vi "MainDAQUse.vi"() -> ()   [LabVIEW 2023]
uses:
  <vilib>/express/express signal manip/GetorSetDDTAttributes/Shared VIs/TimeType.ctl
  <vilib>/DAQmx/read.llb/DAQmx Read (Analog 2D DBL NChan NSamp).vi
  5948bca3-3d14-40bf-9fbb-2ba5c3eee3bd.vi
  <vilib>/Analysis/baseanly.llb/Mean (DBL).vi
  faa81322-6883-41b3-8229-1eb533283c0b.vi
  <extravilib>/ChannelInstances/Tag-bool/Read With Abort.vi
  <extravilib>/ChannelInstances/Tag-bool/Write With Abort.vi
  <extravilib>/ChannelInstances/Tag-bool/Instantiate.vi
  <vilib>/DAQmx/miscellaneous.llb/DAQmx Fill In Error Info.vi
  <extravilib>/ChannelInstances/Tag-bool/EndpointRead.vi
  <vilib>/express/express signal manip/GetorSetDDTAttributes/Shared VIs/TimeMode Enum to Boolean.vi
  <vilib>/express/express shared/transition.llb/Dynamic To Waveform Array.vi
  <vilib>/express/express signal manip/GetorSetDDTAttributes/Set DDT Attributes/SetT0.vi
  <vilib>/express/express shared/transition.llb/Waveform Array To Dynamic.vi
  <extravilib>/ChannelInstances/Tag-bool/Endpoint.vi
  <vilib>/express/express signal manip/GetorSetDDTAttributes/Set DDT Attributes/Set DDT Properties.xnode
  <extravilib>/ChannelInstances/Tag-bool.lvlib
  <vilib>/ptbypt/NI_PtbyPt.lvlib
  <vilib>/Analysis/NI_AALBase.lvlib
  <vilib>/express/express signal manip/GetorSetDDTAttributes/Shared VIs/GetSetShared.lvlib
panel:
  out "Prueba de frecuencia":dynamicdata(graph)
  out "Array":dbl[][](array[numeric])
  out "dt":dbl
  in  "?":T1(tab)
  out "Valor numérico voltaje ACS sin offset":dbl
  out "Signal Frequency":dbl(graph)
  out "Stable RPM measurement?":bool
  in  "R de carga [Ohm]":dbl
  in  "Omega Nominal [RPM]":dbl
  in  "Voltage Threshold":dbl=0.5
  in  "Number of magnets":dbl=1.0
  out "Omega [RPM]":dbl(knob) scale=0.0..2000.0
  out "Voltaje Diodo RMS [V]":dbl(knob) scale=0.0..20.0
  out "Potencia [W]":dbl(knob) scale=0.0..20.0
  out "Voltaje ACS RMS [V]":dbl(knob) scale=0.0..20.0
  in  "Button":bool
  out "Signal\nFrequency (Hz)":dbl
  in  "?":bool
  in  "Button 2":bool
  out "Python Error Status":errorcluster
  in  "Filename":path=path "C:/Users/johan/OneDrive - Estudiantes ITCR/TEC/ProyectodeGraduacion/LabEolicaControl/rawdata.txt"
  out "Corriente ACS RMS [mA]":dbl(knob) scale=0.0..20.0
  out "Valor numérico\nCorriente [mA]":dbl
  out "V Gen RMS [V]":dbl(knob) scale=0.0..20.0
  in  "R1 [Ohm]":dbl=1.0
  in  "R2 [Ohm]":dbl=1.0
  in  "Offset del ACS [V]":dbl=1.0
  in  "Sensibilidad ACS [mV/A]":dbl=1.0
  out "Voltaje diodo [V]":dynamicdata(graph)
  out "Sensor ACS [V]":dynamicdata(graph)
  out "Senal Pulsos":dynamicdata(graph)
  out "Sensor Hall [V]":dynamicdata(graph)
  # "Lab Setup"
  # "Data Monitoring"
  # "Datos para el DAQ"
  # "Condiciones del punto de medida"
  # "File I/O"
  # "Post Processing"
  # "About:"
  # "Software Requirements:"
  # "This measuring system was designed for data acquisition of \npower, angular speed, and resistance data for small scale HAWT \nand possibly VAWT. These turbines are being researched and \ndeveloped at LIENE (Laboratorio de Investigación en Energía Eólica) \nat ITCR. \n\nThis software acquires data and performs post processing to obtain \npower graphs and surfaces and data tables for further analysis. It uses \nLabView for DAQ and integrated Python scripts to post process and \ngraph data."
  # "Python 3.6 with the following packages:\n-- NumPy\n-- Plotly"
  # "Programmer:"
  # "This software was designed and programmed by: \n-- Johansell Villalobos Cubillo & Mauricio Bolivar Gonzalez: \n         Engineering Physics students"
  # "DAQ Equipment: NI-USB-6000"
  # "The equipment pinout diagram is shown below and the pins are used as follows: \n\nAl 0 -- Hall effect sensor\nAl 1-- Voltage sensor\nAl 2 -- ACS712 10A current sensor\nAl GND -- common ground"
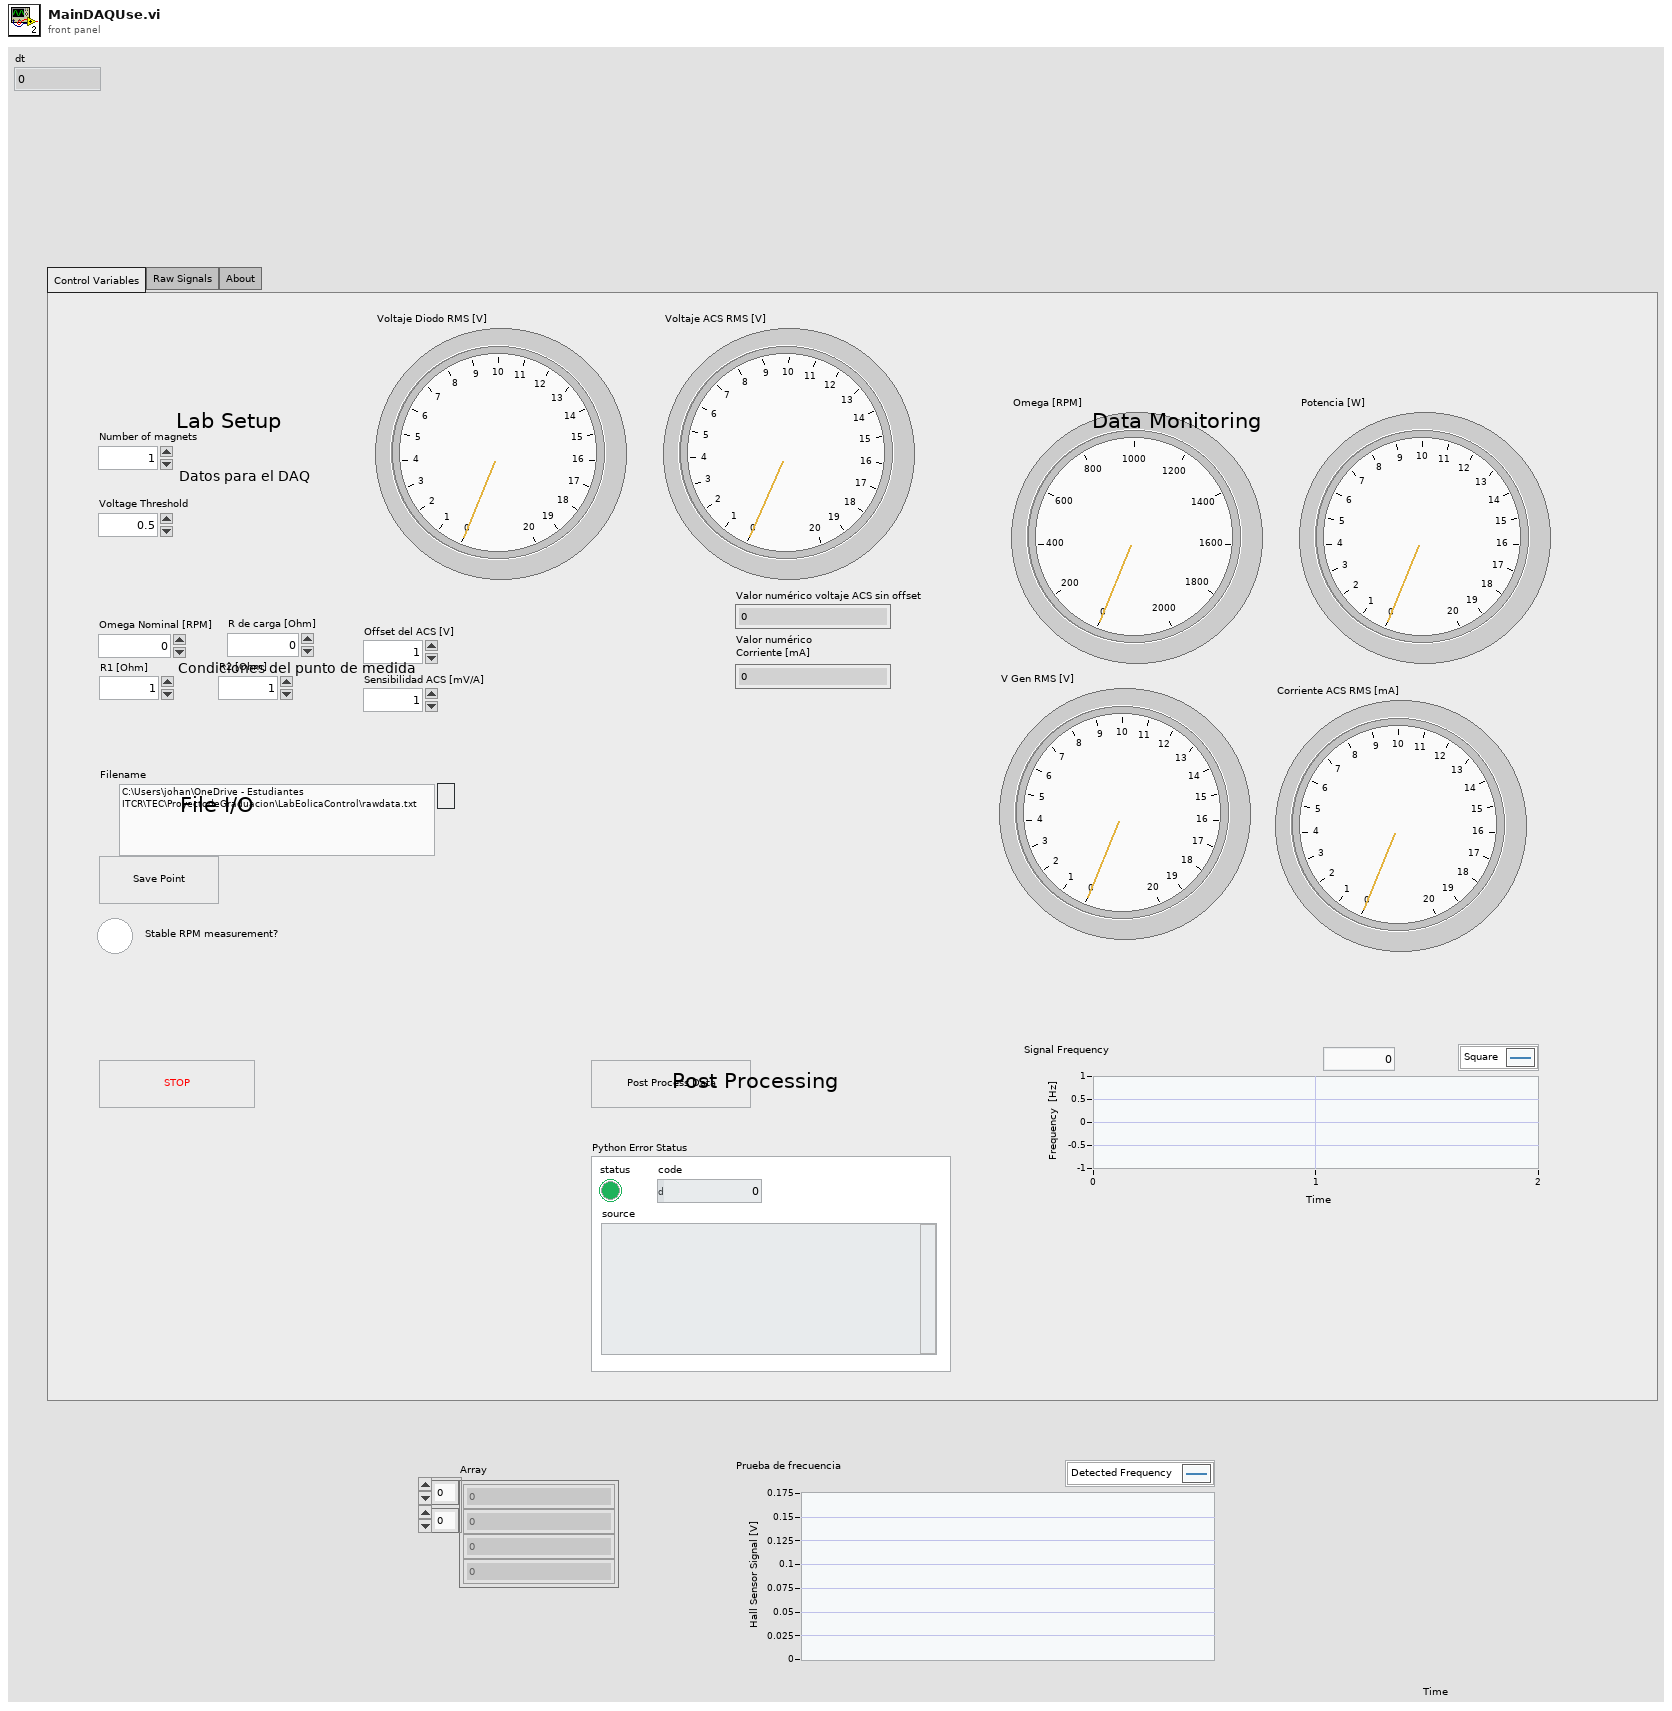
[diagram p1: front panel]
types:
  T1 = enum32{"Control Variables", "Raw Signals", "About"}
  T2 = typedef "Tag-bool.lvlib/))Channel.ctl" = refnum<queue>
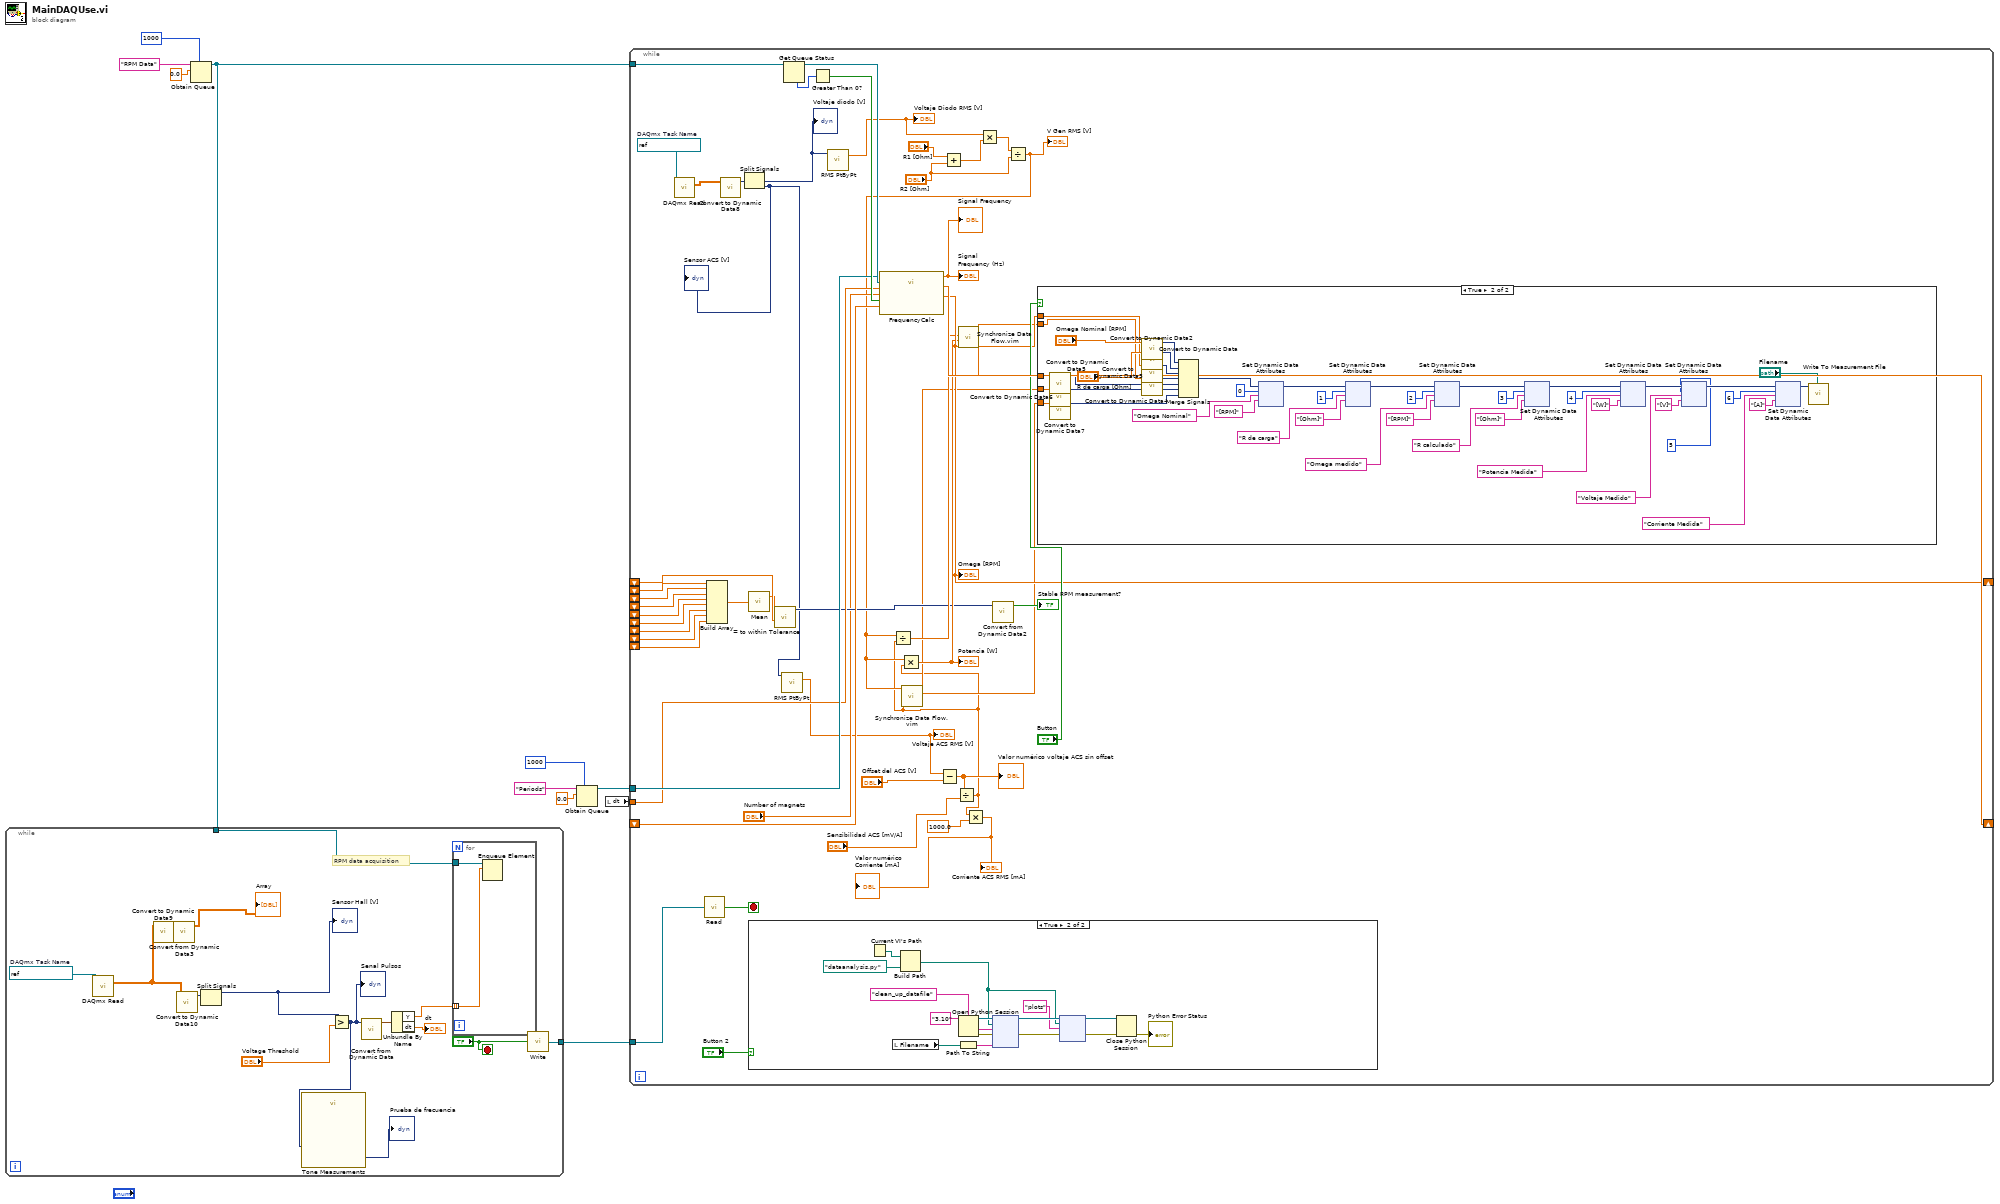
[diagram p0: block diagram]
diagram:
  n1 = Obtain Queue(max queue size (-1, unlimited)=1000 ("max queue size\n(-1, unlimited)"), name (unnamed)="RPM Data" ("name\n(unnamed)"), element data type=0.0 ("data type\n(double)")) -> (queue out=w5:refnum<queue>)  [unwired: 2 in, 2 out]
  n2 = while {
    tunnel: w5 -> [w23]
    tunnel: [w21] -> w7
    stop <- "?" stop-if-true
    w17 = refnum<k21> "DAQ ACS2_0"  # DAQmx Task Name
    # "RPM data acquisition"
    n3 = call-poly <vilib>:"DAQmx Read.vi"("task/channels in"=w17) -> ("data"=w14:dbl[][])  [unwired: 12 in, 2 out]
    n4 = call "Convert to Dynamic Data9"("2D Array"=w14) -> ("Dynamic Data Type"=w16:dynamicdata)  [unwired: 3 in]
    n5 = call "Convert from Dynamic Data3"("Dynamic Data Type"=w16) -> ("Array"=→"Array":dbl[][])  [unwired: 3 in]
    n6 = call "Convert to Dynamic Data10"("2D Array"=w14) -> ("Dynamic Data Type"=w15:dynamicdata)  [unwired: 3 in]
    n7 = Split Signals(w15) -> (w12:dynamicdata)  [unwired: 3 in, 2 out]
    "Sensor Hall [V]" <- w12
    n8 = Greater?(x=w12, y="Voltage Threshold") -> (0:w11:dynamicdata)
    "Senal Pulsos" <- w11
    n9 = call "Tone Measurements"("Signals"=w11) -> ("Frequency"=→"Prueba de frecuencia":dynamicdata)  [unwired: 9 in, 1 out]
    n10 = call "Convert from Dynamic Data"("Dynamic Data Type"=w11) -> ("Waveform"=w25:waveform(dbl))  [unwired: 3 in]
    n11 = Unbundle By Name(w25) -> ("Y"=w24:dbl[], "dt"=→"dt":dbl)
    n12 = for {
      tunnel: w24 -> [w27] mode=indexing
      tunnel: w23 -> [w26]
      n13 = Enqueue Element(queue=w26, element=w27) -> ()  [unwired: 2 in, 3 out]
    }
    n14 = call <extravilib>:"Write.vi"("element"="?") -> ("channel"=w21:T2)  [unwired: 1 out]
  }
  n15 = Obtain Queue(max queue size (-1, unlimited)=1000 ("max queue size\n(-1, unlimited)"), name (unnamed)="Periods" ("name\n(unnamed)"), element data type=0.0 ("data type\n(double)")) -> (queue out=w1:refnum<queue>)  [unwired: 2 in, 2 out]
  n16 = local read "dt"() -> (w6:dbl)
  n17 = while {
    tunnel: w5 -> [w79]
    tunnel: w1 -> [w76]
    shift-right: [w74] -> _
    shift-left: _ -> [w75]
    tunnel: w6 -> [w71]
    tunnel: w7 -> [w72]
    shift-right: [w69] -> _
    shift-left: _ -> [w63]
    shift-left: _ -> [w64]
    shift-left: _ -> [w65]
    shift-left: _ -> [w66]
    shift-left: _ -> [w61]
    shift-left: _ -> [w52]
    shift-left: _ -> [w51]
    shift-left: _ -> [w50]
    shift-left: _ -> [w49]
    stop <- w73 stop-if-true
    w45 = refnum<k21> "DAQ ACS2_0"  # DAQmx Task Name
    n18 = call-poly <vilib>:"DAQmx Read.vi"("task/channels in"=w45) -> ("data"=w44:dbl[][])  [unwired: 12 in, 2 out]
    n19 = call <extravilib>:"Read.vi"("channel"=w72) -> ("element"=w73:bool)  [unwired: 1 in, 1 out]
    n20 = Build Array(w66, w65, w64, w63, w52, w51, w50, w49) -> (w62:dbl[])
    n21 = call "Convert to Dynamic Data8"("2D Array"=w44) -> ("Dynamic Data Type"=w42:dynamicdata)  [unwired: 3 in]
    n22 = Split Signals(w42) -> (w41:dynamicdata, w43:dynamicdata)  [unwired: 3 in, 1 out]
    "Sensor ACS [V]" <- w43
    "Voltaje diodo [V]" <- w41
    n23 = call-poly <vilib>:"Mean.vi"("X"=w62) -> ("mean"=w60:dbl)  [unwired: 1 out]
    n24 = case shown="True" "Button 2" {
      frame False {
      }
      frame True {
        n25 = Current VI's Path() -> (path=w88:path)
        n26 = local read "Filename"() -> (w91:path)
        n27 = Build Path(base path=w88, name or relative path=path "dataanalysis.py") -> (appended path=w85:path)
        n28 = Path To String(path=w91) -> (string=w92:string)
        n29 = Open Python Session(python version="3.10" ("Python version")) -> (session out=w93:refnum<k35>, error out=w94:errorcluster)  [unwired: 2 in]
        n30 = node(w93, w85, "clean_up_datafile" ("function name"), w94, w92) -> (w86:refnum<k35>, w83:errorcluster)  [unwired: 3 in, 2 out]
        n31 = node(w86, w85, "plots" ("function name"), w83) -> (w81:refnum<k35>, w82:errorcluster)  [unwired: 2 in, 2 out]
        n32 = Close Python Session(session in=w81, error in=w82) -> (11:→"Python Error Status":errorcluster)
      }
    }
    n33 = call "= to within Tolerance"("Constant Value to Compare Against"=w61, "Operand 1"=w60) -> ("Result"=w59:dynamicdata)  [unwired: 8 in, 1 out]
    n34 = call <vilib>:"RMS PtByPt.vi"("x"=w43) -> ("rms value"=w40:dbl)  [unwired: 3 in, 1 out]
    "Voltaje ACS RMS [V]" <- w40
    n35 = Get Queue Status(queue=w79) -> (queue out=w77:refnum<queue>, # elements in queue=w80:i32)  [unwired: 2 in, 6 out]
    n36 = Greater Than 0?(x=w80) -> (x > 0?=w78:bool)
    n37 = call <vilib>:"RMS PtByPt.vi"("x"=w41) -> ("rms value"=w30:dbl)  [unwired: 3 in, 1 out]
    "Voltaje Diodo RMS [V]" <- w30
    n38 = call "FrequencyCalc.vi"("Checkbox"=w78, "Number of teeth in gear"="Number of magnets", "Period\n(s) in"=w75, "dt"=w71, "queue in"=w77, "Queue in"=w76) -> ("Omega [RPM]"=w69:dbl, "Period\n(s) out"=w74:dbl, "Signal Frequency (Hz)"=→"Signal\nFrequency (Hz)" →"Signal Frequency":dbl)  [unwired: 2 in, 1 out]
    "Omega [RPM]" <- w69
    n39 = Subtract(x=w40, y="Offset del ACS [V]") -> (x-y=w37:dbl)
    "Valor numérico voltaje ACS sin offset" <- w37
    n40 = Add(x="R1 [Ohm]", y="R2 [Ohm]") -> (x+y=w34:dbl)
    n41 = Divide(x=w37, y="Sensibilidad ACS [mV/A]") -> (x/y=w28:dbl)
    n42 = Multiply(x=w28, y=1000.0) -> (x*y=→"Corriente ACS RMS [mA]" →"Valor numérico\nCorriente [mA]":dbl)
    n43 = Multiply(x=w30, y=w34) -> (x*y=w36:dbl)
    n44 = call "Convert from Dynamic Data2"("Dynamic Data Type"=w59) -> ("Scalar"=→"Stable RPM measurement?":bool)  [unwired: 3 in]
    n45 = Divide(x=w36, y="R2 [Ohm]") -> (x/y=w29:dbl)
    "V Gen RMS [V]" <- w29
    n46 = Divide(x=w29, y=w28) -> (x/y=w68:dbl)
    n47 = Multiply(x=w29, y=w28) -> (x*y=w67:dbl)
    "Potencia [W]" <- w67
    n48 = call "Synchronize Data Flow.vim"("input 2"=w28, "input 1"=w29) -> ("output 2"=w46:dbl, "output 1"=w47:dbl)  [unwired: 2 in, 2 out]
    n49 = call "Synchronize Data Flow.vim"("input 4"=w69, "input 3"=w67, "input 2"=w68) -> ("output 4"=w57:dbl, "output 3"=w55:dbl, "output 2"=w56:dbl)  [unwired: 1 in, 1 out]
    n50 = case shown="True" "Button" {
      tunnel: w57 -> [_ w134]
      tunnel: w56 -> [_ w135]
      tunnel: w55 -> [_ w130]
      tunnel: w47 -> [_ w108]
      tunnel: w46 -> [_ w107]
      frame False {
      }
      frame True {
        n51 = call "Convert to Dynamic Data5"("Double"=w130) -> ("Dynamic Data Type"=w131:dynamicdata)  [unwired: 3 in]
        n52 = call "Convert to Dynamic Data6"("Double"=w108) -> ("Dynamic Data Type"=w106:dynamicdata)  [unwired: 3 in]
        n53 = call "Convert to Dynamic Data7"("Double"=w107) -> ("Dynamic Data Type"=w105:dynamicdata)  [unwired: 3 in]
        n54 = call "Convert to Dynamic Data"("Double"="Omega Nominal [RPM]") -> ("Dynamic Data Type"=w137:dynamicdata)  [unwired: 3 in]
        n55 = call "Convert to Dynamic Data2"("Double"="R de carga [Ohm]") -> ("Dynamic Data Type"=w136:dynamicdata)  [unwired: 3 in]
        n56 = call "Convert to Dynamic Data3"("Double"=w134) -> ("Dynamic Data Type"=w133:dynamicdata)  [unwired: 3 in]
        n57 = call "Convert to Dynamic Data4"("Double"=w135) -> ("Dynamic Data Type"=w132:dynamicdata)  [unwired: 3 in]
        n58 = Merge Signals(w137, w136, w133, w132, w131, w106, w105) -> (w129:dynamicdata)
        n59 = xnode ("Set Dynamic Data Attributes")("Signals In"=w129, "Signal Index"=0, "Signal Name"="Omega Nominal", "Unit"="[RPM]") -> ("Signals Out"=w122:dynamicdata)  [unwired: 3 in, 1 out]
        n60 = xnode ("Set Dynamic Data Attributes")("Signals In"=w122, "Signal Index"=1, "Signal Name"="R de carga", "Unit"="[Ohm]") -> ("Signals Out"=w118:dynamicdata)  [unwired: 3 in, 1 out]
        n61 = xnode ("Set Dynamic Data Attributes")("Signals In"=w118, "Signal Index"=2, "Signal Name"="Omega medido", "Unit"="[RPM]") -> ("Signals Out"=w114:dynamicdata)  [unwired: 3 in, 1 out]
        n62 = xnode ("Set Dynamic Data Attributes")("Signals In"=w114, "Signal Index"=3, "Signal Name"="R calculado", "Unit"="[Ohm]") -> ("Signals Out"=w110:dynamicdata)  [unwired: 3 in, 1 out]
        n63 = xnode ("Set Dynamic Data Attributes")("Signals In"=w110, "Signal Index"=4, "Signal Name"="Potencia Medida", "Unit"="[W]") -> ("Signals Out"=w98:dynamicdata)  [unwired: 3 in, 1 out]
        n64 = xnode ("Set Dynamic Data Attributes")("Signals In"=w98, "Signal Index"=5, "Signal Name"="Voltaje Medido", "Unit"="[V]") -> ("Signals Out"=w100:dynamicdata)  [unwired: 3 in, 1 out]
        n65 = xnode ("Set Dynamic Data Attributes")("Signals In"=w100, "Signal Index"=6, "Signal Name"="Corriente Medida", "Unit"="[A]") -> ("Signals Out"=w97:dynamicdata)  [unwired: 3 in, 1 out]
        n66 = call "Write To Measurement File"("Signals"=w97, "Filename"="Filename") -> ()  [unwired: 15 in, 3 out]
      }
    }
  }
